vi "Trigger Detector (DBL).vi"(0 "data in":dbl, 1 "reset? (F)":bool, 5 "trigger definition":T3, 9 "data timestamp":timestamp, 11 "error in (no error)":errorcluster) -> (4 "triggers":T1(array[cluster]), 6 "actual trigger state":T2, 15 "error out":errorcluster)   [LabVIEW 2014, in "NI_EP_Power Quality.lvlib"]
doc: "Detects crossing of limits for the measurement that you specify and returns triggers if occur.\n\nThis VI supports measuring single-line and multiple-line systems except the DBL instance. Use the DBL instance to measure one channel on one line at one time."
uses:
  <vilib>/addons/Electrical Power/PQ/NI_EP_Power Quality.lvlib
  <vilib>/addons/Electrical Power/PQ/Common/Controls/ep_Trigger State.ctl
  <vilib>/addons/Electrical Power/PQ/Triggers/subVIs/ep_Trigger Definition.ctl
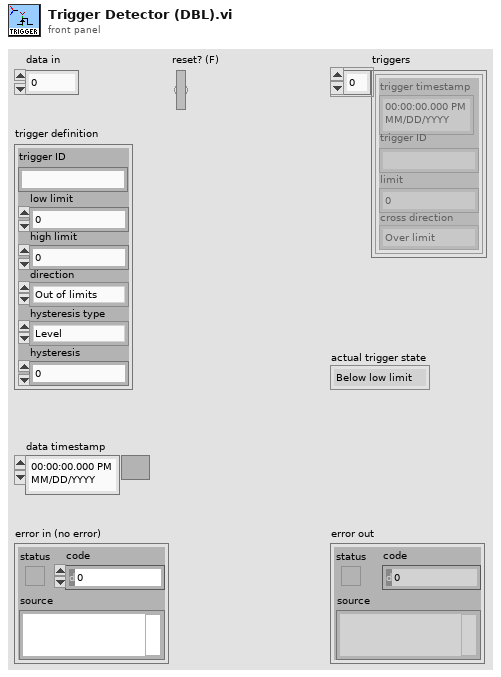
[diagram p1: front panel]
types:
  T1 = cluster{"trigger timestamp":timestamp, "trigger ID":string, "limit":dbl, "cross direction":enum16{"Over limit", "Below limit"}}[]
  T2 = typedef "NI_EP_Power Quality.lvlib/ep_Trigger State.ctl" = enum16{"Below low limit", "In the limits", "Over high limit"}
  T3 = cluster{"trigger ID":string, "low limit":dbl, "high limit":dbl, "direction":enum16{"Out of limits", "Back to limits", "Both"}, "hysteresis type":enum16{"Level", "Time"}, "hysteresis":dbl}
  T4 = typedef "NI_EP_Power Quality.lvlib/ep_Trigger Definition.ctl" = cluster{"trigger ID":string, "low limit":dbl, "high limit":dbl, "direction":enum16{"Out of limits", "Back to limits", "Both"}, "hysteresis type":enum16{"Level", "Time"}, "hysteresis":dbl}
  T5 = cluster{"Lo in progr.":bool, "Hi in progr.":bool, "Lo trig. time":timestamp, "Hi trig. time":timestamp}
  T6 = enum16{"Out of limits", "Back to limits", "Both"}
  T7 = cluster{"Lo in progr.":bool, "Lo in progr.":bool, "data timestamp":timestamp, "data timestamp":timestamp}
  T8 = cluster{"trigger time":timestamp, "trigger unique id":string, "limit":dbl, "cross direction":enum16{"Over limit", "Below limit"}}[]
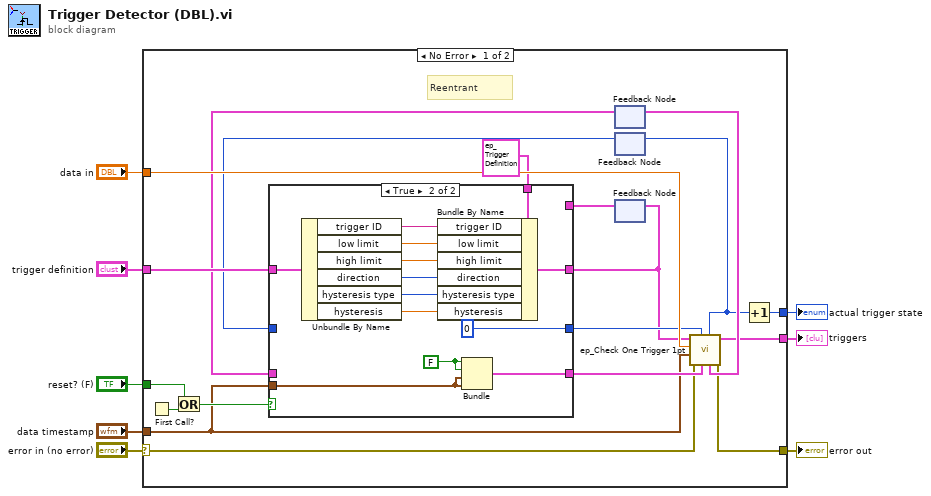
[diagram p0: block diagram]
diagram:
  n1 = case shown="No Error" "error in (no error)" {
    selector: "error in (no error)" -> [w13 w44]
    tunnel: "data in" -> [w27 _]
    tunnel: "reset? (F)" -> [w25 _]
    tunnel: "trigger definition" -> [w23 _]
    tunnel: "data timestamp" -> [w14 _]
    tunnel: [w12 w44] -> w8
    tunnel: [w10 _] -> w2
    tunnel: [w9 _] -> w1
    frame No Error {
      # "Reentrant"
      n2 = First Call?() -> (First Call?: T/F=w26:bool)
      n3 = Or(x=w25, y=w26) -> (x .or. y?=w24:bool)
      n4 = feedback #1() -> (w17:T5)  [unwired: 1 in]
      n5 = feedback #2() -> (w19:i8)  [unwired: 1 in]
      n6 = feedback #3() -> (w16:T4)  [unwired: 1 in]
      n7 = case shown="True" w24 {
        tunnel: w23 -> [_ w43]
        tunnel: [w28 w42] -> w15
        tunnel: T4 {"trigger ID"="", "low limit"=0.0, "high limit"=0.0, "direction"=enum."Out of limits", "hysteresis type"=enum."Level", "hysteresis"=0.0} ("trigger definition") -> [_ w41]
        tunnel: [w30 w40] -> w21
        tunnel: [w29 i8 0] -> w20
        tunnel: w19 -> [w29 _]
        tunnel: w17 -> [w30 _]
        tunnel: w16 -> [w28 _]
        tunnel: w14 -> [_ w38]
        frame False {
        }
        frame True {
          w33 = FALSE ("Lo in progr.")
          n8 = Unbundle By Name(w43) -> ("trigger ID"=w36:string, "low limit"=w32:dbl, "high limit"=w31:dbl, "direction"=w35:T6, "hysteresis type"=w34:enum16{"Level", "Time"}, "hysteresis"=w37:dbl)
          n9 = Bundle By Name(cluster=w41, "trigger ID"=w36, "low limit"=w32, "high limit"=w31, "direction"=w35, "hysteresis type"=w34, "hysteresis"=w37) -> (w42:T4)
          n10 = Bundle("Lo in progr."=w33, "Lo in progr."=w33, "data timestamp"=w38, "data timestamp"=w38) -> (w40:T7)  [unwired: 1 in]
        }
      }
      n11 = feedback-in #3(w15) -> ()
      n12 = call <vilib>:"ep_Check One Trigger 1pt.vi"("trig. local in"=w21, "prev. state in"=w20, "error in (no error)"=w13, "data time stamp"=w14, "value in"=w27, "trigger definition"=w15) -> ("error out"=w12:errorcluster, "triggers list"=w9:T8, "trig. local out"=w18:T5, "state out"=w11:i8)  [unwired: 2 in]
      n13 = feedback-in #1(w18) -> ()
      n14 = feedback-in #2(w11) -> ()
      n15 = Increment(x=w11) -> (x+1=w10:i8)
    }
    frame Error {
    }
  }
  "error out" <- w8
  "actual trigger state" <- w2
  "triggers" <- w1
